vi "Schematic.vi"() -> ()   [LabVIEW 2011]
uses:
  GlobalVariables.vi
panel:
  in  "26":bool caption="49"
  in  "111":bool caption="49"
  out "Ion Guage":dbl format="%#_5e"
  out "GP275 Conv.":sgl format="%#_5e"
  in  "Open (100)":bool
  in  "Close (99)":bool
  in  "105":bool caption="49"
  in  "107":bool caption="49"
  in  "117":bool caption="49"
  in  "109":bool caption="49"
  in  "101":bool caption="49"
  in  "115":bool caption="49"
  in  "TV":bool caption="49"
  in  "110":bool caption="49"
  in  "103":bool caption="49"
  out "BAR 95":dbl format="%#_5e"
  out "BAR 94":dbl format="%#_5e"
  out "BAR 93":dbl format="%#_3e"
  out "BAR 92":dbl format="%#_3e"
  out "BAR 91":dbl format="%#_4e"
  out "BAR 90":dbl format="%#_4e"
  in  "RTPC 27":dbl
  out "RTPC 27":dbl
  in  "RTPC 30":dbl
  out "RTPC 30":dbl=34.586588541666664
  in  "PC 0000000000":dbl
  in  "MFC 74":dbl
  in  "MFC 73":dbl
  out "PC 0000000000":dbl
  out "MFC 74":dbl
  out "MFC 73":dbl
  in  "MFC 83":dbl
  in  "MFC 82":dbl
  in  "MFC 81":dbl
  out "MFC 83":dbl
  out "MFC 82":dbl
  out "MFC 81":dbl
  in  "MFC 80":dbl
  in  "MFC 79":dbl
  in  "MFC 78":dbl
  out "MFC 80":dbl
  out "MFC 79":dbl
  out "MFC 78":dbl
  in  "MFC 86":dbl
  in  "MFC 85":dbl
  in  "MFC 84":dbl
  out "MFC 86":dbl
  out "MFC 85":dbl
  out "MFC 84":dbl
  in  "MFC 70":dbl
  in  "MFC 69":dbl
  in  "MFC 68":dbl
  out "MFC 70":dbl
  out "MFC 69":dbl
  out "MFC 68":dbl
  in  "PC 43":dbl
  out "PC 43":dbl
  in  "MFC 36":dbl
  in  "MFC 38":dbl
  out "MFC 36":dbl
  out "MFC 38":dbl
  in  "MFC 39":dbl
  in  "PC 42":dbl
  in  "MFC 35":dbl
  in  "MFC 34":dbl
  out "MFC 39":dbl
  out "PC 42":dbl
  out "MFC 35":dbl
  out "MFC 34":dbl
  in  "PC 24":dbl
  in  "MFC 23":dbl
  in  "PC 21":dbl
  in  "MFC 20":dbl
  out "PC 24":dbl
  out "MFC 23":dbl
  out "PC 21":dbl
  out "MFC 20":dbl
  in  "MFC 22":dbl
  in  "MFC 33":dbl
  in  "MFC 32":dbl
  in  "MFC 19":dbl
  out "MFC 22":dbl
  out "MFC 33":dbl
  out "MFC 32":dbl
  out "MFC 19":dbl
  in  "19":bool caption="49"
  in  "20":bool caption="49"
  in  "29":bool caption="49"
  in  "53":bool caption="49"
  in  "54":bool caption="49"
  in  "55":bool caption="49"
  in  "77":bool caption="49"
  in  "78":bool caption="49"
  in  "79":bool caption="49"
  in  "80":bool caption="49"
  in  "56":bool caption="49"
  in  "81":bool caption="49"
  in  "84":bool caption="49"
  in  "24":bool caption="49"
  in  "24":bool caption="49"
  in  "Flip 91/92":bool
  in  "RTPC 27":dbl
  out "RTPC 27":dbl
  in  "RTPC 28":dbl
  out "RTPC 28":dbl=34.586588541666664
  in  "Flip 33/34":bool
  in  "Flip 35/36":bool
  in  "Flip 37/38":bool
  in  "Flip 49/50":bool
  in  "Flip 39/40":bool
  in  "Flip 45/46":bool
  in  "Flip 47/48":bool
  in  "Flip 41/42":bool
  in  "Flip 43/44":bool
  in  "MFC 57":dbl
  out "MFC 57":dbl
  in  "23":bool caption="49"
  in  "25":bool caption="49"
  in  "MFC 41":dbl
  out "MFC 41":dbl
  in  "76":bool caption="49"
  in  "75":bool caption="49"
  in  "66":bool caption="49"
  in  "65":bool caption="49"
  in  "68":bool caption="49"
  in  "67":bool caption="49"
  in  "70":bool caption="49"
  in  "69":bool caption="49"
  in  "72":bool caption="49"
  in  "71":bool caption="49"
  in  "74":bool caption="49"
  in  "73":bool caption="49"
  in  "38":bool caption="49"
  in  "37":bool caption="49"
  in  "50":bool caption="49"
  in  "49":bool
  in  "52":bool caption="49"
  in  "51":bool caption="49"
  in  "36":bool caption="49"
  in  "35":bool caption="49"
  in  "34":bool caption="49"
  in  "33":bool caption="49"
  in  "MFC ? 70":dbl
  in  "PC 17":dbl
  in  "MFC 54":dbl
  in  "MFC 54":dbl
  in  "MFC 08":dbl
  in  "PC 16":dbl
  in  "MFC 53":dbl
  in  "MFC 52":dbl
  in  "MFC 07":dbl
  in  "PC 15":dbl
  in  "MFC 51":dbl
  in  "MFC 50":dbl
  in  "MFC 06":dbl
  in  "PC 14":dbl
  in  "MFC 49":dbl
  in  "MFC 48":dbl
  in  "MFC 05":dbl
  in  "PC 13":dbl
  in  "MFC 04":dbl
  in  "MFC 56":dbl
  in  "MFC 37":dbl
  out "MFC ? 71":dbl
  out "PC 17":dbl
  out "MFC 54":dbl
  out "MFC 54":dbl
  out "MFC 08":dbl
  in  "PC 12":dbl
  in  "MFC 03":dbl
  in  "MFC 47":dbl
  in  "PC 11":dbl
  in  "MFC 02":dbl
  in  "MFC 46":dbl
  in  "RTPC 28":dbl
  in  "MFC 45":dbl
  in  "MFC 44":dbl
  in  "MFC 01":dbl
  out "PC 16":dbl
  out "MFC 53":dbl
  out "MFC 52":dbl
  out "MFC 07":dbl
  out "PC 15":dbl
  out "MFC 51":dbl
  out "MFC 50":dbl
  out "MFC 06":dbl
  out "PC 14":dbl
  out "MFC 49":dbl
  out "MFC 48":dbl
  out "MFC 05":dbl
  out "PC 13":dbl
  out "MFC 04":dbl
  out "MFC 56":dbl
  out "MFC 37":dbl
  out "PC 12":dbl
  out "MFC 03":dbl
  out "MFC 47":dbl
  out "PC 11":dbl
  out "MFC 02":dbl
  out "MFC 46":dbl
  out "RTPC 28":dbl
  out "MFC 45":dbl
  out "MFC 44":dbl
  out "MFC 01":dbl
  in  "07":bool caption="49"
  in  "08":bool caption="49"
  in  "08":bool caption="49"
  in  "17":bool caption="49"
  in  "18":bool caption="49"
  in  "18":bool caption="49"
  in  "64":bool caption="49"
  in  "15":bool caption="49"
  in  "16":bool caption="49"
  in  "16":bool caption="49"
  in  "63":bool caption="49"
  in  "13":bool caption="49"
  in  "14":bool caption="49"
  in  "14":bool caption="49"
  in  "62":bool caption="49"
  in  "11":bool caption="49"
  in  "12":bool caption="49"
  in  "12":bool caption="49"
  in  "22":bool caption="49"
  in  "21":bool caption="49"
  in  "22":bool caption="49"
  in  "61":bool caption="49"
  in  "09":bool caption="49"
  in  "57":bool caption="49"
  in  "05":bool caption="49"
  in  "10":bool caption="49"
  in  "10":bool caption="49"
  in  "58":bool caption="49"
  in  "58":bool caption="49"
  in  "06":bool caption="49"
  in  "06":bool caption="49"
  in  "90":bool caption="49"
  in  "03":bool caption="49"
  in  "04":bool caption="49"
  in  "04":bool caption="49"
  in  "01":bool caption="49"
  in  "02":bool caption="49"
  in  "02":bool caption="49"
  in  "59":bool caption="49"
  in  "27":bool caption="49"
  in  "30":bool caption="49"
  in  "94":bool caption="49"
  in  "93":bool caption="49"
  in  "?":bool caption="49"
  in  "28":bool caption="49"
  in  "31":bool caption="49"
  in  "95":bool caption="49"
  in  "96":bool caption="49"
  in  "90":bool caption="49"
  in  "92":bool caption="49"
  in  "91":bool caption="49"
  in  "86":bool caption="49"
  in  "85":bool caption="49"
  in  "48":bool caption="49"
  in  "47":bool caption="49"
  in  "46":bool caption="49"
  in  "45":bool caption="49"
  in  "44":bool caption="49"
  in  "43":bool caption="49"
  in  "42":bool caption="49"
  in  "41":bool caption="49"
  in  "40":bool caption="49"
  in  "39":bool caption="49"
  in  "CloseVi?":bool=TRUE
  in  "Close":bool
  # "19"
  # "20"
  # "32"
  # "21"
  # "33"
  # "23"
  # "22"
  # "24"
  # "34"
  # "35"
  # "38"
  # "42"
  # "36"
  # "39"
  # "19"
  # "20"
  # "Arsine"
  # "32"
  # "21"
  # "H2"
  # "33"
  # "23"
  # "AsH3 1-DD VENT"
  # "22"
  # "AsH3 2-DD VENT"
  # "24"
  # "Si2H6 DD VENT"
  # "34"
  # "30"
  # "HYDRIDE GROWTH"
  # "Phosphine"
  # "35"
  # "30"
  # "38"
  # "42"
  # "HYDRIDE VENT"
  # "29"
  # "73"
  # "74"
  # "75"
  # "29"
  # "?"
  # "36"
  # "TO SHROUD"
  # "39"
  # "TO PURGE"
  # "81"
  # "82"
  # "83"
  # "73"
  # "74"
  # "78"
  # "79"
  # "80"
  # "75"
  # "57"
  # "86"
  # "85"
  # "84"
  # "28"
  # "81"
  # "ALKYL GROWTH"
  # "82"
  # "ALKYL VENT"
  # "68"
  # "69"
  # "70"
  # "27"
  # "83"
  # "78"
  # "ALKYL DD VENT"
  # "79"
  # "57"
  # "80"
  # "28"
  # "09"
  # "08"
  # "54"
  # "07"
  # "52"
  # "06"
  # "50"
  # "05"
  # "48"
  # "04"
  # "37"
  # "56"
  # "03"
  # "46"
  # "02"
  # "01"
  # "44"
  # "84"
  # "27"
  # "55"
  # "17"
  # "53"
  # "16"
  # "51"
  # "15"
  # "49"
  # "14"
  # "13"
  # "43"
  # "12"
  # "11"
  # "47"
  # "45"
  # "10"
  # "85"
  # "VACUUM"
  # "86"
  # "VENT"
  # "68"
  # "69"
  # "TMAl #2"
  # "70"
  # "DMHy"
  # "TMAl #1"
  # "TMGa #2"
  # "TMGa #1"
  # "TMIn #2"
  # "Spare"
  # "TMIn #1"
  # "CCl4"
  # "DEZn"
  # "07"
  # "01"
  # "03"
  # "04"
  # "09"
  # "52"
  # "12"
  # "44"
  # "13"
  # "53"
  # "45"
  # "05"
  # "46"
  # "37"
  # "16"
  # "10"
  # "48"
  # "02"
  # "56"
  # "08"
  # "06"
  # "49"
  # "11"
  # "41"
  # "43"
  # "54"
  # "50"
  # "14"
  # "47"
  # "55"
  # "51"
  # "41"
  # "17"
  # "15"
  # "TO GLOVE BOX"
  # "N2"
  # "TO TURBO PUMP"
  # "TO EBARA"
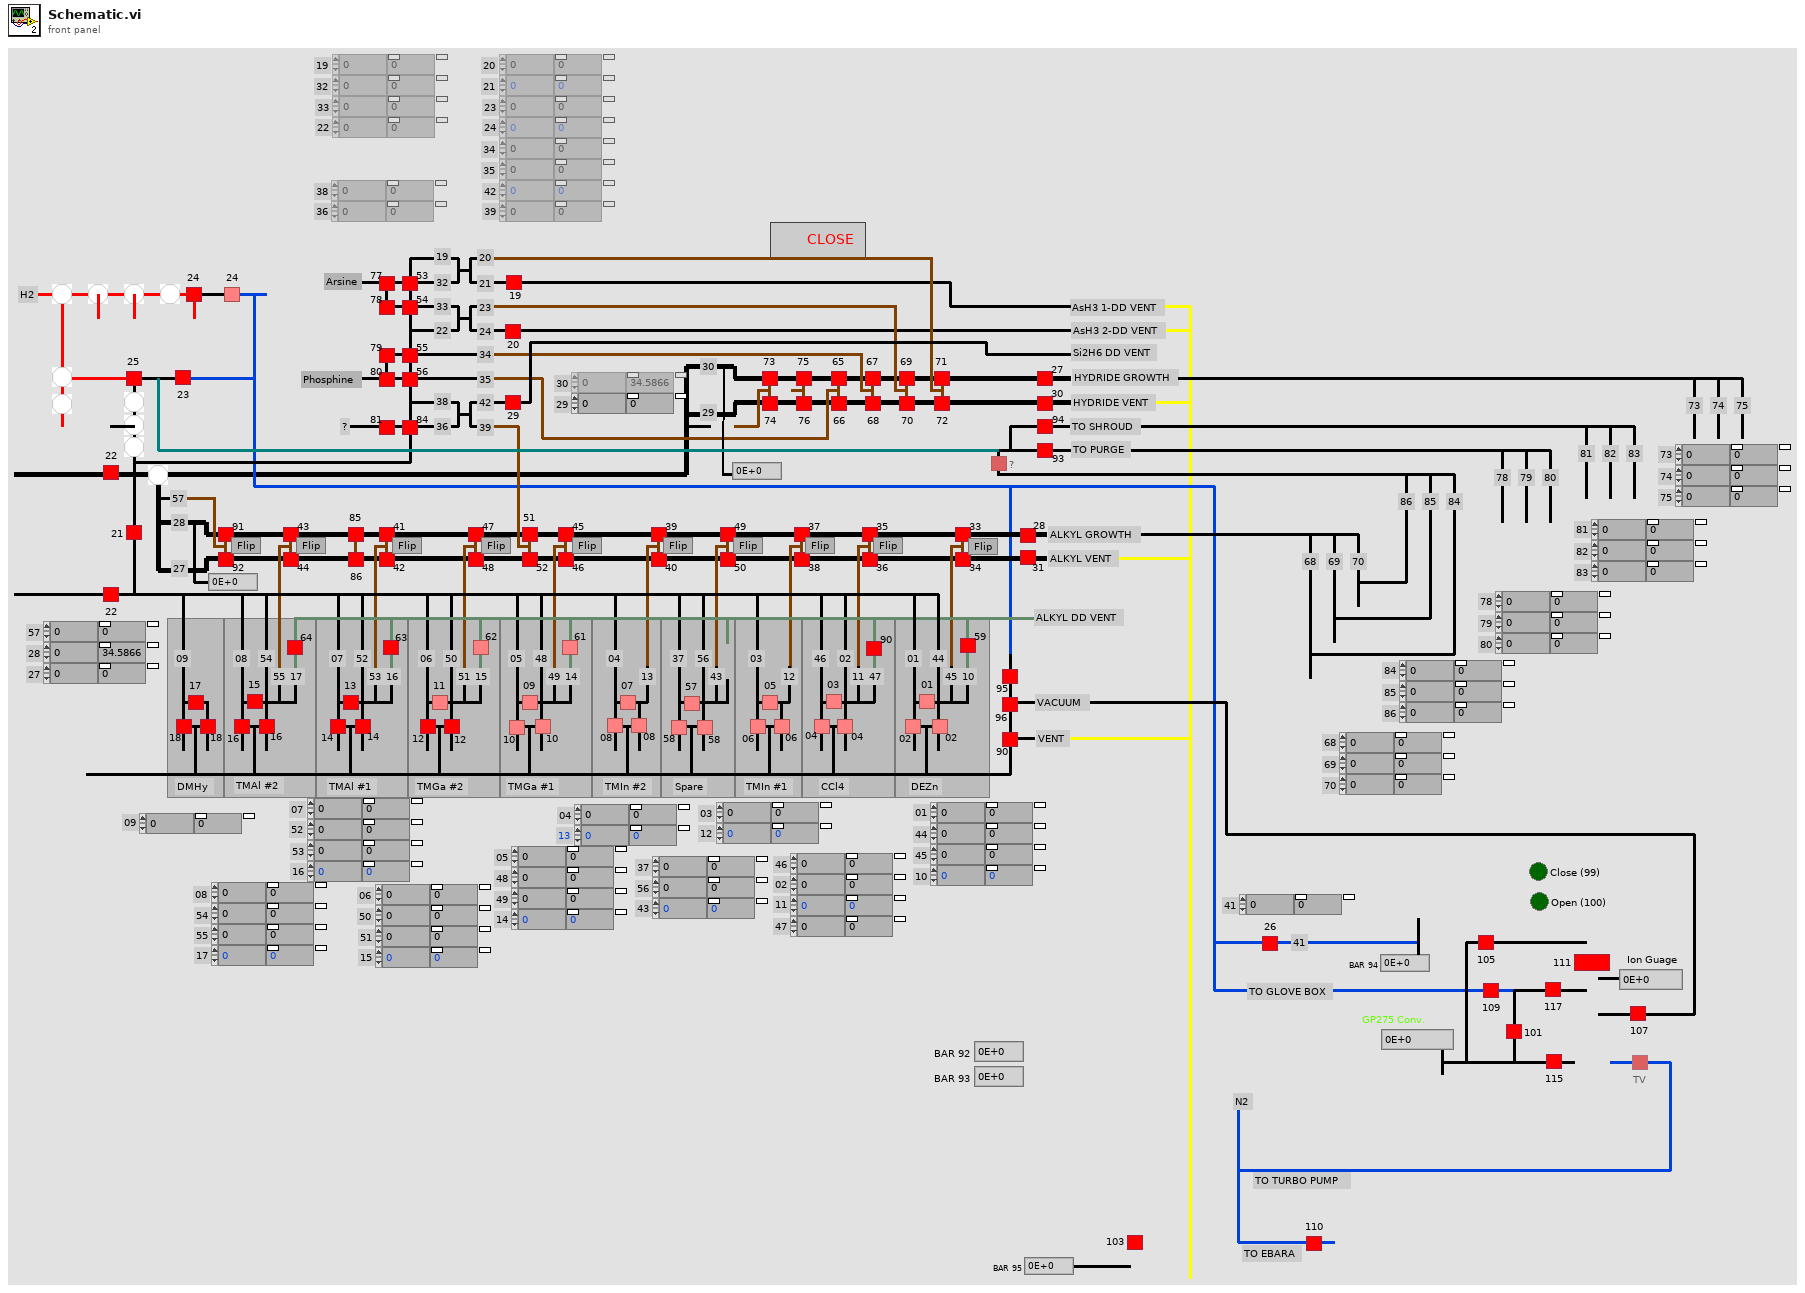
[diagram p1: front panel]
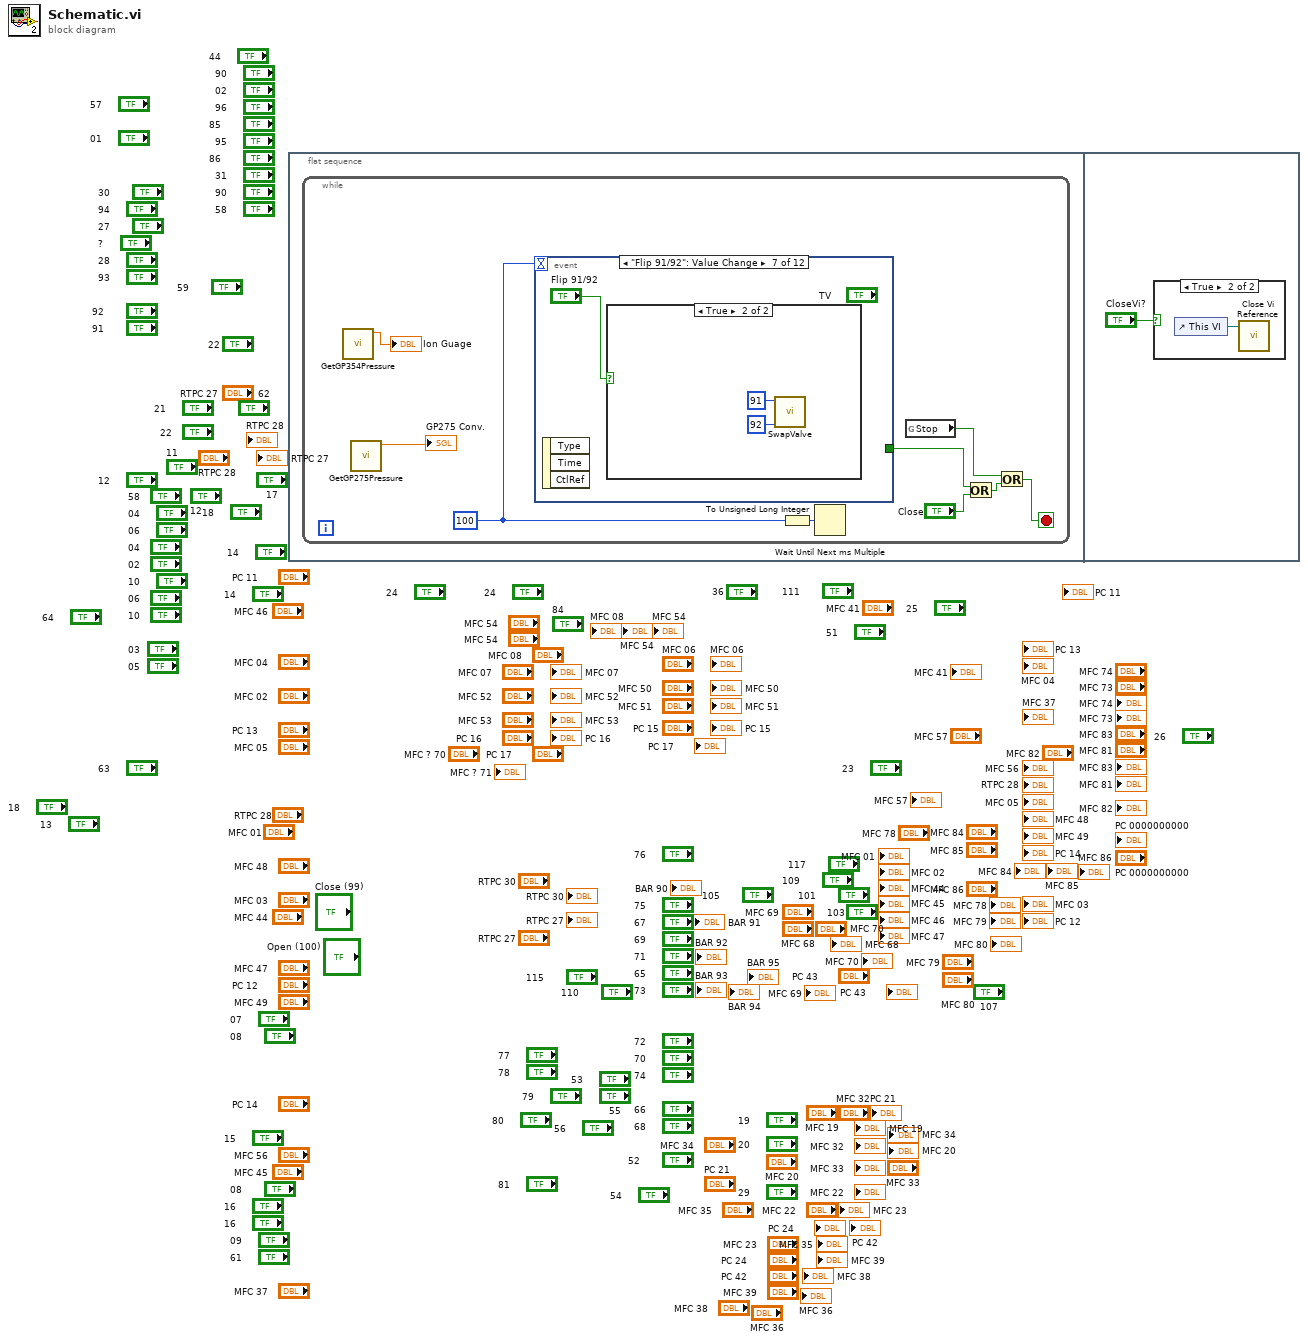
[diagram p0: block diagram]
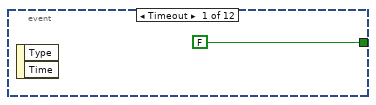
[diagram p2: hidden frame]
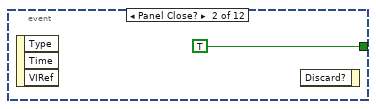
[diagram p3: hidden frame]
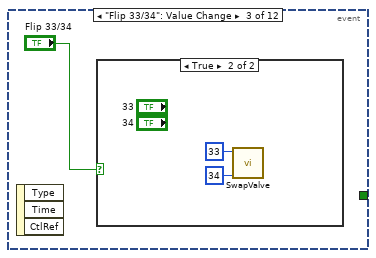
[diagram p4: hidden frame]
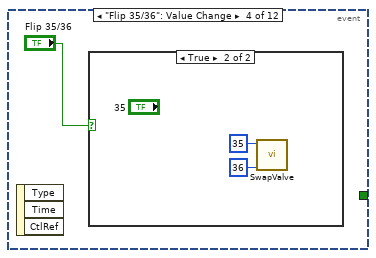
[diagram p6: hidden frame]
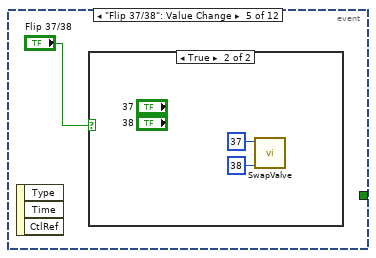
[diagram p8: hidden frame]
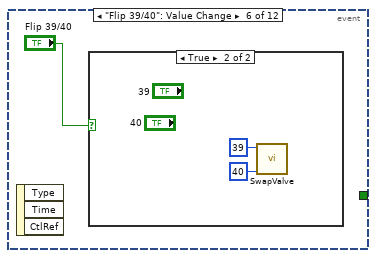
[diagram p10: hidden frame]
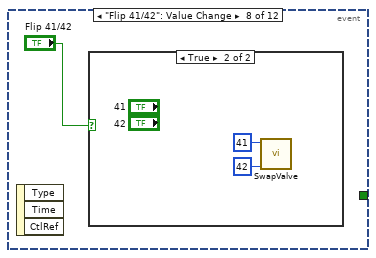
[diagram p13: hidden frame]
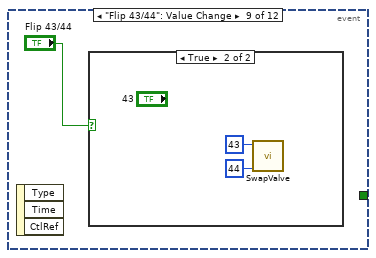
[diagram p15: hidden frame]
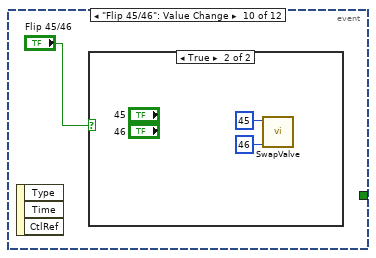
[diagram p17: hidden frame]
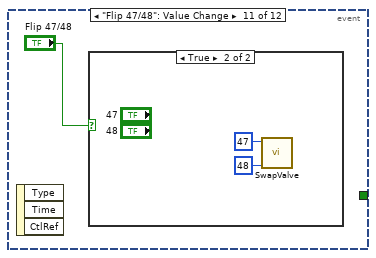
[diagram p19: hidden frame]
diagram:
  n1 = flat-sequence {
    frame #0 {
      n2 = while {
        stop <- w3 stop-if-true
        w4 = 100
        n3 = call "GetGP354Pressure.vi"() -> ("Pressure"=→"Ion Guage":dbl)  [unwired: 11 in]
        n4 = call "GetGP275Pressure.vi"() -> ("Pressure (Torr)"=→"GP275 Conv.":sgl)  [unwired: 11 in]
        n5 = event shown="[6] \"Flip 91/92\": Value Change" {
          selector: _ -> [_ _ _ _ _ _ _ _ _ _ _ _]
          dyn-events: _ -> [_ _ _ _ _ _ _ _ _ _ _ _]
          timeout: w4 -> [_ _ _ _ _ _ _ _ _ _ _ _]
          tunnel: [FALSE ("y") TRUE ("y") _ _ _ _ _ _ _ _ _ _] -> w6
          event Timeout {
            n6 = event-data() -> ()  [unwired: 1 in, 2 out]
          }
          event Panel Close? {
            n7 = event-data() -> ()  [unwired: 1 in, 3 out]
            n8 = event-data() -> ()  [unwired: 2 in, 1 out]
          }
          event "Flip 33/34": Value Change {
            n9 = event-data() -> ()  [unwired: 1 in, 3 out]
            n10 = case shown="True" "Flip 33/34" {
              frame False {
              }
              frame True {
                n11 = call "SwapValve.vi"("Valve 2"=34, "Valve 1"=33) -> ()  [unwired: 10 in]
              }
            }
          }
          event "Flip 35/36": Value Change {
            n12 = event-data() -> ()  [unwired: 1 in, 3 out]
            n13 = case shown="True" "Flip 35/36" {
              frame False {
              }
              frame True {
                n14 = call "SwapValve.vi"("Valve 2"=36, "Valve 1"=35) -> ()  [unwired: 10 in]
              }
            }
          }
          event "Flip 37/38": Value Change {
            n15 = event-data() -> ()  [unwired: 1 in, 3 out]
            n16 = case shown="True" "Flip 37/38" {
              frame False {
              }
              frame True {
                n17 = call "SwapValve.vi"("Valve 2"=38, "Valve 1"=37) -> ()  [unwired: 10 in]
              }
            }
          }
          event "Flip 39/40": Value Change {
            n18 = event-data() -> ()  [unwired: 1 in, 3 out]
            n19 = case shown="True" "Flip 39/40" {
              frame False {
              }
              frame True {
                n20 = call "SwapValve.vi"("Valve 2"=40, "Valve 1"=39) -> ()  [unwired: 10 in]
              }
            }
          }
          event "Flip 91/92": Value Change {
            n21 = event-data() -> ()  [unwired: 1 in, 3 out]
            n22 = case shown="True" "Flip 91/92" {
              frame False {
              }
              frame True {
                n23 = call "SwapValve.vi"("Valve 2"=92, "Valve 1"=91) -> ()  [unwired: 10 in]
              }
            }
          }
          event "Flip 41/42": Value Change {
            n24 = event-data() -> ()  [unwired: 1 in, 3 out]
            n25 = case shown="True" "Flip 41/42" {
              frame False {
              }
              frame True {
                n26 = call "SwapValve.vi"("Valve 2"=42, "Valve 1"=41) -> ()  [unwired: 10 in]
              }
            }
          }
          event "Flip 43/44": Value Change {
            n27 = event-data() -> ()  [unwired: 1 in, 3 out]
            n28 = case shown="True" "Flip 43/44" {
              frame False {
              }
              frame True {
                n29 = call "SwapValve.vi"("Valve 2"=44, "Valve 1"=43) -> ()  [unwired: 10 in]
              }
            }
          }
          event "Flip 45/46": Value Change {
            n30 = event-data() -> ()  [unwired: 1 in, 3 out]
            n31 = case shown="True" "Flip 45/46" {
              frame False {
              }
              frame True {
                n32 = call "SwapValve.vi"("Valve 2"=46, "Valve 1"=45) -> ()  [unwired: 10 in]
              }
            }
          }
          event "Flip 47/48": Value Change {
            n33 = event-data() -> ()  [unwired: 1 in, 3 out]
            n34 = case shown="True" "Flip 47/48" {
              frame False {
              }
              frame True {
                n35 = call "SwapValve.vi"("Valve 2"=48, "Valve 1"=47) -> ()  [unwired: 10 in]
              }
            }
          }
          event "Flip 49/50": Value Change {
            n36 = event-data() -> ()  [unwired: 1 in, 3 out]
            n37 = case shown="True" "Flip 49/50" {
              frame False {
              }
              frame True {
                n38 = call "SwapValve.vi"("Valve 2"=50, "Valve 1"=49) -> ()  [unwired: 10 in]
              }
            }
          }
        }
        n39 = To Unsigned Long Integer(number=w4) -> (unsigned 32bit integer=w5:u32)
        n40 = Wait Until Next ms Multiple(millisecond multiple=w5) -> ()  [unwired: 1 out]
        n41 = global read "GlobalVariables.vi" "Stop"() -> (w9:bool)
        n42 = Or(x=w6, y="Close") -> (x .or. y?=w8:bool)
        n43 = Or(x=w9, y=w8) -> (x .or. y?=w3:bool)
      }
    }
    frame #1 {
      n44 = case shown="True" "CloseVi?" {
        frame False {
        }
        frame True {
          n45 = control-ref of="This VI"() -> (w43:refnum<vi>)
          n46 = call "Close Vi Reference.vi"("reference"=w43) -> ()  [unwired: 9 in, 2 out]
        }
      }
    }
  }
